vi "Convert_C_to_F.vi"(1 "deg C":dbl) -> (0 "deg F":dbl)   [LabVIEW 2023]
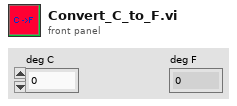
[diagram p1: front panel]
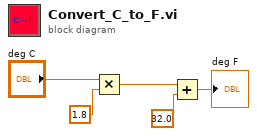
[diagram p0: block diagram]
diagram:
  n1 = Multiply(x="deg C", y=1.8) -> (x*y=w2:dbl)
  n2 = Add(x=w2, y=32.0) -> (x+y=→"deg F":dbl)
